vi "GetState.vi"(8 "error in (no error)":errorcluster, 11 "SMO":refnum<class "SMO.lvclass">) -> (0 "error out":errorcluster, 2 "SMO State":T1, 3 "SMO out":refnum<class "SMO.lvclass">)   [LabVIEW 2019, in "SMO.lvclass"]
doc: "JKI State Machine Objects (SMO) 1.3.0.56\nJKI - JKI\nCopyright (c) 2017, JKI"
uses:
  SMO.lvclass
  Typedefs/SMOState --Enum.ctl
panel:
  # "For instructions on how to use the JKI State Machine Objects, examples and video tutorials, visit:\nhttp://jki.net/state-machine-objects/\n\nJKI State Machine Objects™\nhttp://jki.net/state-machine-objects/\nCopyright (C) 2005-2015, JKI <info@jki.net>\nALL RIGHTS RESERVED"
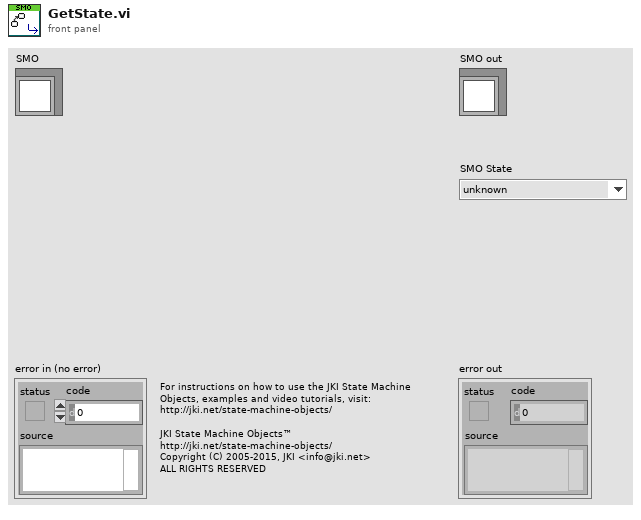
[diagram p1: front panel]
types:
  T1 = typedef "SMO.lvclass/SMOState --Enum.ctl" = enum16{"unknown", "Created", "Started", "Stopped"}
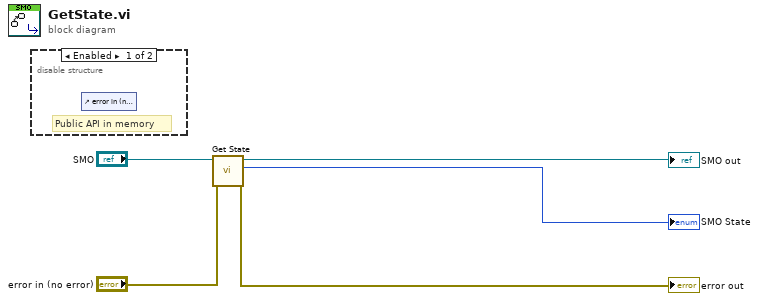
[diagram p0: block diagram]
diagram:
  n1 = disable-structure shown="Enabled" {
    frame Enabled {
      # "Public API in memory"
      n2 = control-ref of="error in (no error)"() -> ()  [unwired: 1 out]
    }
    frame Disabled {
    }
  }
  n3 = call "Get State.vi"("error in (no error)"="error in (no error)", "SMO"="SMO") -> ("error out"=→"error out":errorcluster, "SMO State"=→"SMO State":T1, "SMO out"=→"SMO out":refnum<class "SMO.lvclass">)  [unwired: 7 in]
